vi "Time.Secs to H_M_S.vi"(11 "Total Secs":dbl format="%#.3f") -> (0 "Secs":dbl, 1 "Mins":dbl, 2 "Hours":dbl, 3 "Duration":string)   [LabVIEW 2018]
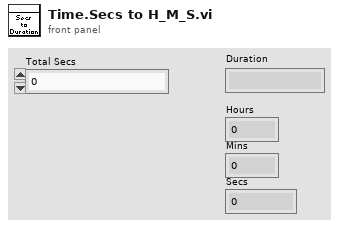
[diagram p1: front panel]
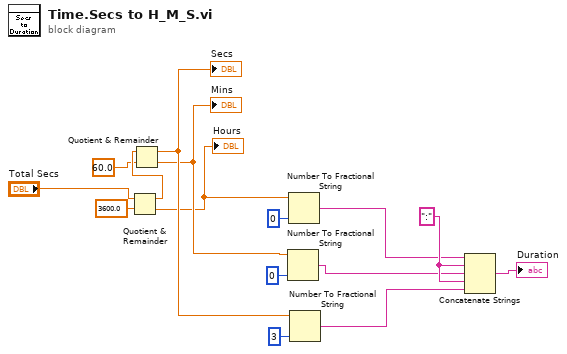
[diagram p0: block diagram]
diagram:
  w5 = ":"
  n1 = Quotient & Remainder(x="Total Secs", y=3600.0) -> (x-y*floor(x/y)=w14:dbl, floor(x/y)=w7:dbl)
  "Hours" <- w7
  n2 = Quotient & Remainder(x=w14, y=60.0) -> (x-y*floor(x/y)=w12:dbl, floor(x/y)=w8:dbl)
  "Mins" <- w8
  "Secs" <- w12
  n3 = Number To Fractional String(number=w8, precision (6)=i16 0) -> (F-format string=w3:string)  [unwired: 2 in]
  n4 = Number To Fractional String(number=w7, precision (6)=i16 0) -> (F-format string=w4:string)  [unwired: 2 in]
  n5 = Number To Fractional String(number=w12, precision (6)=i16 3) -> (F-format string=w2:string)  [unwired: 2 in]
  n6 = Concatenate Strings(w4, w5, w3, w5, w2) -> (→"Duration":string)
